vi "NewBallLifetime.vi"(10 "last balls":refnum<class "Ball.lvclass">[](array[class]), 11 "Balls":refnum<class "Ball.lvclass">[](array[class])) -> (3 "balls out":refnum<class "Ball.lvclass">[](array[class]))   [LabVIEW 2018]
uses:
  Ball_class/Ball.lvclass
  Ball_class/Ball.lvclass/Ball.ctl
  Ball_class/Write Valid.vi
panel:
  in  "Life Time":dbl=2.0
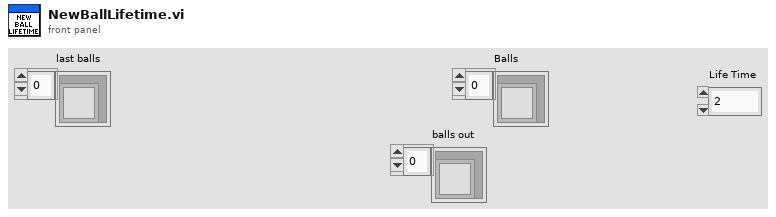
[diagram p1: front panel]
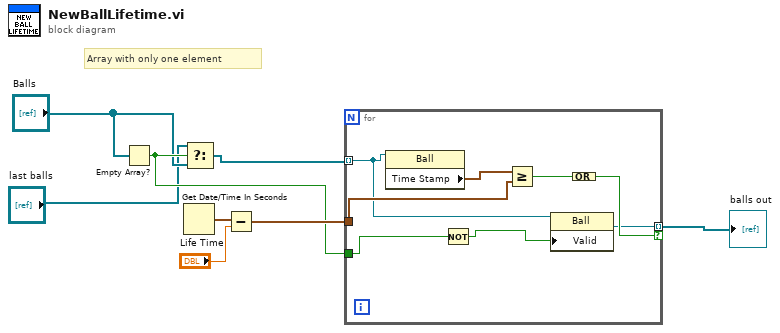
[diagram p0: block diagram]
diagram:
  # "Array with only one element"
  n1 = Empty Array?(array="Balls") -> (empty?=w4:bool)
  n2 = Get Date/Time In Seconds() -> (seconds since 1Jan1904=w8:timestamp)
  n3 = Select(t="last balls", s=w4, f="Balls") -> (s? t:f=w5:refnum<class "Ball.lvclass">[])
  n4 = Subtract(x=w8, y="Life Time") -> (x-y=w6:timestamp)
  n5 = for {
    tunnel: w5 -> [w11] mode=indexing
    tunnel: [w9] -> w1 mode=indexing if=w16
    tunnel: w6 -> [w14]
    tunnel: w4 -> [w13]
    n6 = property class="Ball"(reference=w11) -> ("Time Stamp"=w12:timestamp)  [unwired: 1 in, 2 out]
    n7 = Not(x=w13) -> (.not. x?=w10:bool)
    n8 = Greater Or Equal?(x=w12, y=w14) -> (x >= y?=w15:bool)
    n9 = property class="Ball"(reference=w11, "Valid"=w10) -> (reference out=w9:refnum<class "Ball.lvclass">)  [unwired: 1 in, 1 out]
    n10 = Compound Arithmetic op=OR(w15) -> (w16:bool)
  }
  "balls out" <- w1
